vi "Read Wear_in.vi"(8 "error in (no error)":errorcluster, 11 "EVI 79 in":refnum<class "EVI 79.lvclass">) -> (0 "error out":errorcluster, 2 "Wear_in":T1={"V"=24.0, "I"=0.5, "Cycles"=0.5, "On_Time_ms"=0.5, "Off_Time_ms"=0.5}, 3 "EVI 79 out":refnum<class "EVI 79.lvclass">)   [LabVIEW 2025, in "EVI 79.lvclass"]
uses:
  EVI 79.lvclass
  EVI 79.lvclass/EVI 79.ctl
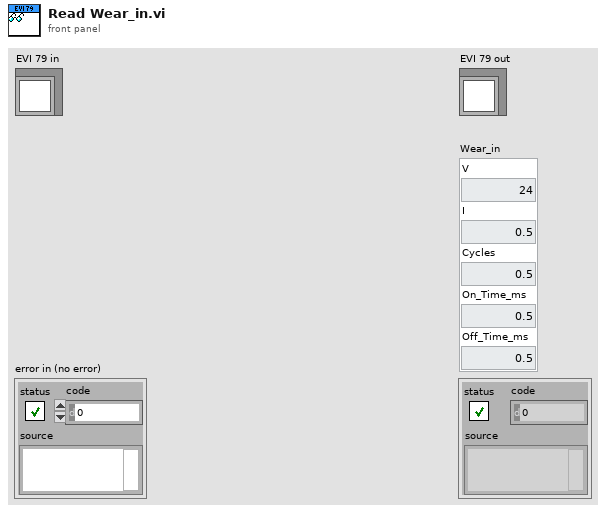
[diagram p1: front panel]
types:
  T1 = cluster{"V":dbl, "I":dbl, "Cycles":dbl, "On_Time_ms":dbl, "Off_Time_ms":dbl}
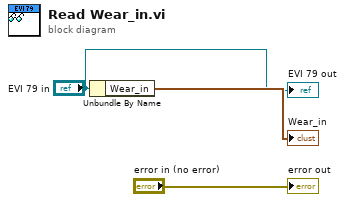
[diagram p0: block diagram]
diagram:
  n1 = Unbundle By Name("EVI 79 in") -> ("Wear_in"=→"Wear_in":T1)
  "error out" <- "error in (no error)"
  "EVI 79 out" <- "EVI 79 in"
